vi "XIPIN_Virtex-6_FPGA_GTH_Transceiver_Wizard_1_11.vi"   [LabVIEW 2017]
doc: "Compatible Production devices only. Use the Virtex-6 FPGA GTH Transceiver Wizard to configure one or more Virtex-6 FPGA GTH transceivers. Start from scratch, or use an industry standard template. The Wizard generates a custom wrapper for the transceivers you've selected. In addition, it produces an example design, testbench, and scripts to allow users to observe the transceivers operating under simulation and in hardware.\n------------------------------------\n<b>Need License</b> : No"
uses:
  <vilib>/rvi/XilinxIP/XIPIN_XNode/niFpgaXIPIN.xnode
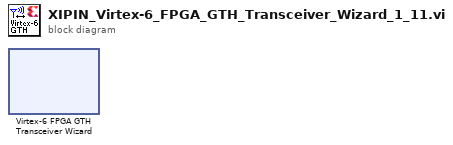
[diagram p0: block diagram]
diagram:
  n1 = xnode ("Virtex-6 FPGA GTH Transceiver Wizard")() -> ()
